vi "Lab Panel V4.88.vi"() -> ()   [LabVIEW 2013] (continued)
                n1776 = property on="O/I  LAB03-2" class="Bool (strict)"("DisabledEnum"=w3326) -> ()  [unwired: 2 in, 2 out]
                n1777 = Not(x=w3331) -> (.not. x?=w3332:bool)
                n1778 = Not(x=w3330) -> (.not. x?=w3333:bool)
                n1779 = Not(x=w3329) -> (.not. x?=w3334:bool)
                n1780 = property on="RESULT LAB05-2" class="Bool (strict)"("Visible"=w3332) -> ()  [unwired: 2 in, 2 out]
                n1781 = property on="RESULT LAB05-1" class="Bool (strict)"("Visible"=w3333) -> ()  [unwired: 2 in, 2 out]
                n1782 = Not(x=w3328) -> (.not. x?=w3335:bool)
                n1783 = property on="RESULT LAB04-2" class="Bool (strict)"("Visible"=w3334) -> ()  [unwired: 2 in, 2 out]
                n1784 = Not(x=w3327) -> (.not. x?=w3336:bool)
                n1785 = property on="RESULT LAB04-1" class="Bool (strict)"("Visible"=w3335) -> ()  [unwired: 2 in, 2 out]
                n1786 = property on="RESULT LAB03-2" class="Bool (strict)"("Visible"=w3336) -> ()  [unwired: 2 in, 2 out]
              }
              frame #2 {
                # "disable calibrate if any test running"
                n1787 = Or(x=w3359, y=w3358) -> (x .or. y?=w3352:bool)
                n1788 = Or(x=w3361, y=w3360) -> (x .or. y?=w3354:bool)
                n1789 = Or(x=w3365, y=w3364) -> (x .or. y?=w3356:bool)
                n1790 = Or(x=w3363, y=w3362) -> (x .or. y?=w3355:bool)
                n1791 = Or(x=w3367, y=w3366) -> (x .or. y?=w3357:bool)
                n1792 = Or(x=w3355, y=w3354) -> (x .or. y?=w3353:bool)
                n1793 = Or(x=w3357, y=w3356) -> (x .or. y?=w3351:bool)
                n1794 = Or(x=w3353, y=w3352) -> (x .or. y?=w3350:bool)
                n1795 = Or(x=w3351, y=w3350) -> (x .or. y?=w3349:bool)
                n1796 = case shown="False" w3349 {
                  tunnel: [0 2] -> w3348
                  frame False {
                  }
                  frame True {
                  }
                }
                n1797 = property on="JIG TEST" class="Clust (strict)"("DisabledEnum"=w3348) -> ()  [unwired: 2 in, 2 out]
                n1798 = property on="Network Directory" class="Path"("DisabledEnum"=w3348) -> ()  [unwired: 2 in, 2 out]
                n1799 = property on="MAIL SETTINGS" class="Clust (strict)"("DisabledEnum"=w3348) -> ()  [unwired: 2 in, 2 out]
                n1800 = property on="SET (cal)" class="Bool (strict)"("DisabledEnum"=w3348) -> ()  [unwired: 2 in, 2 out]
                n1801 = property on="ADMIN" class="Bool (strict)"("DisabledEnum"=0) -> ()  [unwired: 2 in, 2 out]
              }
            }
          }
          frame #8 {
            # "drive jigs"
            n1802 = stacked-sequence {
              frame #0 {
                # "jig on"
                n1803 = local read "jig cycle"() -> (w3375:dbl)
                n1804 = property on="JIG TEST" class="Clust (strict)"() -> ("DisabledEnum"=w3372:T16)  [unwired: 2 in, 2 out]
                n1805 = Equal?(x=w3372, y=2) -> (x = y?=w3371:bool)
                n1806 = Equal?(x=w3375, y=0) -> (x = y?=w3373:bool)
                n1807 = And(x=w3373, y=w3371) -> (x .and. y?=w3370:bool)
                n1808 = case shown="True" w3370 {
                  frame False {
                  }
                  frame True {
                    n1809 = local read "run lab01-1"() -> (w3386:bool)
                    n1810 = local read "run lab01-2"() -> (w3385:bool)
                    n1811 = local read "run lab02-1"() -> (w3384:bool)
                    n1812 = local read "run lab02-2"() -> (w3383:bool)
                    n1813 = local read "run lab03-1"() -> (w3382:bool)
                    n1814 = local read "run lab03-2"() -> (w3381:bool)
                    n1815 = local read "run lab04-1"() -> (w3380:bool)
                    n1816 = local read "run lab04-2"() -> (w3379:bool)
                    n1817 = local read "run lab05-1"() -> (w3378:bool)
                    n1818 = local read "run lab05-2"() -> (w3377:bool)
                    n1819 = local write "JIG LAB03-2"(w3381) -> ()
                    n1820 = local write "JIG LAB01-1"(w3386) -> ()
                    n1821 = local write "JIG LAB01-2"(w3385) -> ()
                    n1822 = local write "JIG LAB02-1"(w3384) -> ()
                    n1823 = local write "JIG LAB02-2"(w3383) -> ()
                    n1824 = local write "JIG LAB03-1"(w3382) -> ()
                    n1825 = local write "JIG LAB04-1"(w3380) -> ()
                    n1826 = local write "JIG LAB04-2"(w3379) -> ()
                    n1827 = local write "JIG LAB05-1"(w3378) -> ()
                    n1828 = local write "JIG LAB05-2"(w3377) -> ()
                  }
                }
              }
              frame #1 {
                # "jig off"
                n1829 = local read "jig cycle"() -> (w3393:dbl)
                n1830 = local read "on loops"() -> (w3392:dbl)
                n1831 = property on="JIG TEST" class="Clust (strict)"() -> ("DisabledEnum"=w3391:T16)  [unwired: 2 in, 2 out]
                n1832 = Equal?(x=w3391, y=2) -> (x = y?=w3389:bool)
                n1833 = Equal?(x=w3393, y=w3392) -> (x = y?=w3388:bool)
                n1834 = And(x=w3388, y=w3389) -> (x .and. y?=w3387:bool)
                n1835 = case shown="True" w3387 {
                  frame False {
                  }
                  frame True {
                    w3444 = FALSE
                    w3445 = TRUE
                    w3443 = 2
                    n1836 = local read "SELECT LAB05-2"() -> (w3434:T3)
                    n1837 = local read "SELECT LAB04-2"() -> (w3436:T3)
                    n1838 = local read "SELECT LAB04-1"() -> (w3437:T3)
                    n1839 = local read "SELECT LAB05-1"() -> (w3435:T3)
                    n1840 = local read "SELECT LAB03-2"() -> (w3438:T3)
                    n1841 = local read "SELECT LAB02-1"() -> (w3441:T3)
                    n1842 = local read "SELECT LAB03-1"() -> (w3439:T3)
                    n1843 = local read "SELECT LAB02-2"() -> (w3440:T3)
                    n1844 = local read "SELECT LAB01-2"() -> (w3442:T3)
                    n1845 = local read "run lab05-1"() -> (w3404:bool)
                    n1846 = local read "run lab05-2"() -> (w3403:bool)
                    n1847 = local read "SELECT LAB01-1"() -> (w3446:T3)
                    n1848 = local read "run lab04-2"() -> (w3405:bool)
                    n1849 = local read "run lab04-1"() -> (w3406:bool)
                    n1850 = local read "run lab01-1"() -> (w3422:bool)
                    n1851 = local read "run lab01-2"() -> (w3411:bool)
                    n1852 = local read "run lab03-2"() -> (w3407:bool)
                    n1853 = local read "run lab03-1"() -> (w3408:bool)
                    n1854 = local read "run lab02-1"() -> (w3410:bool)
                    n1855 = local read "run lab02-2"() -> (w3409:bool)
                    n1856 = Equal?(x=w3443, y=w3439) -> (x = y?=w3417:bool)
                    n1857 = Equal?(x=w3443, y=w3438) -> (x = y?=w3416:bool)
                    n1858 = Equal?(x=w3443, y=w3437) -> (x = y?=w3415:bool)
                    n1859 = Equal?(x=w3443, y=w3436) -> (x = y?=w3414:bool)
                    n1860 = Equal?(x=w3443, y=w3435) -> (x = y?=w3413:bool)
                    n1861 = Equal?(x=w3443, y=w3434) -> (x = y?=w3412:bool)
                    n1862 = Equal?(x=w3443, y=w3446) -> (x = y?=w3423:bool)
                    n1863 = Equal?(x=w3443, y=w3441) -> (x = y?=w3419:bool)
                    n1864 = Equal?(x=w3443, y=w3440) -> (x = y?=w3418:bool)
                    n1865 = Equal?(x=w3443, y=w3442) -> (x = y?=w3420:bool)
                    n1866 = And(x=w3414, y=w3405) -> (x .and. y?=w3396:bool)
                    n1867 = And(x=w3417, y=w3408) -> (x .and. y?=w3399:bool)
                    n1868 = And(x=w3415, y=w3406) -> (x .and. y?=w3397:bool)
                    n1869 = And(x=w3412, y=w3403) -> (x .and. y?=w3394:bool)
                    n1870 = And(x=w3418, y=w3409) -> (x .and. y?=w3400:bool)
                    n1871 = And(x=w3416, y=w3407) -> (x .and. y?=w3398:bool)
                    n1872 = And(x=w3413, y=w3404) -> (x .and. y?=w3395:bool)
                    n1873 = And(x=w3420, y=w3411) -> (x .and. y?=w3402:bool)
                    n1874 = And(x=w3423, y=w3422) -> (x .and. y?=w3421:bool)
                    n1875 = And(x=w3419, y=w3410) -> (x .and. y?=w3401:bool)
                    n1876 = Select(t=w3445, s=w3421, f=w3444) -> (s? t:f=w3424:bool)
                    n1877 = Select(t=w3445, s=w3402, f=w3444) -> (s? t:f=w3425:bool)
                    n1878 = Select(t=w3445, s=w3401, f=w3444) -> (s? t:f=w3426:bool)
                    n1879 = Select(t=w3445, s=w3400, f=w3444) -> (s? t:f=w3427:bool)
                    n1880 = Select(t=w3445, s=w3399, f=w3444) -> (s? t:f=w3428:bool)
                    n1881 = Select(t=w3445, s=w3398, f=w3444) -> (s? t:f=w3429:bool)
                    n1882 = Select(t=w3445, s=w3397, f=w3444) -> (s? t:f=w3430:bool)
                    n1883 = Select(t=w3445, s=w3396, f=w3444) -> (s? t:f=w3431:bool)
                    n1884 = Select(t=w3445, s=w3395, f=w3444) -> (s? t:f=w3432:bool)
                    n1885 = Select(t=w3445, s=w3394, f=w3444) -> (s? t:f=w3433:bool)
                    n1886 = local write "JIG LAB03-2"(w3429) -> ()
                    n1887 = local write "JIG LAB02-1"(w3426) -> ()
                    n1888 = local write "JIG LAB02-2"(w3427) -> ()
                    n1889 = local write "JIG LAB01-2"(w3425) -> ()
                    n1890 = local write "JIG LAB03-1"(w3428) -> ()
                    n1891 = local write "JIG LAB01-1"(w3424) -> ()
                    n1892 = local write "JIG LAB05-2"(w3433) -> ()
                    n1893 = local write "JIG LAB04-1"(w3430) -> ()
                    n1894 = local write "JIG LAB05-1"(w3432) -> ()
                    n1895 = local write "JIG LAB04-2"(w3431) -> ()
                  }
                }
              }
            }
          }
          frame #9 {
            # "enable  jig test output if no test busy"
            n1896 = property on="JIG TEST" class="Clust (strict)"() -> ("DisabledEnum"=w3449:T16)  [unwired: 2 in, 2 out]
            n1897 = Equal?(x=w3449, y=0) -> (x = y?=w3447:bool)
            n1898 = case shown="True" w3447 {
              frame False {
              }
              frame True {
                n1899 = local read "JIG TEST"() -> (w3460:T10)
                n1900 = Unbundle(w3460) -> ("LAB01-1"=w3459:bool, "LAB01-2"=w3458:bool, "LAB02-1"=w3457:bool, "LAB02-2"=w3456:bool, "LAB03-1"=w3455:bool, "LAB03-2"=w3454:bool, "LAB04-1"=w3453:bool, "LAB04-2"=w3452:bool, "LAB05-1"=w3451:bool, "LAB05-2"=w3450:bool)
                n1901 = local write "JIG LAB05-1"(w3451) -> ()
                n1902 = local write "JIG LAB05-2"(w3450) -> ()
                n1903 = local write "JIG LAB04-1"(w3453) -> ()
                n1904 = local write "JIG LAB04-2"(w3452) -> ()
                n1905 = local write "JIG LAB03-2"(w3454) -> ()
                n1906 = local write "JIG LAB01-1"(w3459) -> ()
                n1907 = local write "JIG LAB02-1"(w3457) -> ()
                n1908 = local write "JIG LAB03-1"(w3455) -> ()
                n1909 = local write "JIG LAB01-2"(w3458) -> ()
                n1910 = local write "JIG LAB02-2"(w3456) -> ()
              }
            }
          }
          frame #10 {
            # "drive digital output"
            n1911 = local read "O/I  LAB05-2"() -> (w3467:bool)
            n1912 = local read "O/I  LAB05-1"() -> (w3469:bool)
            n1913 = local read "JIG LAB05-2"() -> (w3466:bool)
            n1914 = local read "O/I  LAB04-2"() -> (w3471:bool)
            n1915 = local read "JIG LAB05-1"() -> (w3468:bool)
            n1916 = local read "JIG LAB04-2"() -> (w3470:bool)
            n1917 = local read "O/I  LAB03-1"() -> (w3476:bool)
            n1918 = local read "O/I  LAB04-1"() -> (w3472:bool)
            n1919 = local read "O/I  LAB02-1"() -> (w3480:bool)
            n1920 = local read "O/I  LAB02-2"() -> (w3478:bool)
            n1921 = local read "O/I  LAB03-2"() -> (w3474:bool)
            n1922 = local read "JIG LAB04-1"() -> (w3465:bool)
            n1923 = local read "JIG LAB03-2"() -> (w3473:bool)
            n1924 = local read "O/I  LAB01-2"() -> (w3482:bool)
            n1925 = local read "JIG LAB02-1"() -> (w3479:bool)
            n1926 = local read "JIG LAB02-2"() -> (w3477:bool)
            n1927 = local read "JIG LAB03-1"() -> (w3475:bool)
            n1928 = local read "O/I  LAB01-1"() -> (w3484:bool)
            n1929 = local read "JIG LAB01-2"() -> (w3481:bool)
            n1930 = local read "JIG LAB01-1"() -> (w3483:bool)
            n1931 = Build Array(w3471, w3470, w3469, w3468, w3467, w3466) -> (w3462:bool[])
            n1932 = Build Array(w3477, w3476, w3475, w3474, w3473, w3472, w3465) -> (w3463:bool[])
            n1933 = Build Array(w3484, w3483, w3482, w3481, w3480, w3479, w3478) -> (w3464:bool[])
            n1934 = local read "simulate"() -> (w3461:bool)
            n1935 = case shown="False" w3461 {
              tunnel: w3464 -> [w3487 _]
              tunnel: w3463 -> [w3486 _]
              tunnel: w3462 -> [w3485 _]
              frame False {
                n1936 = call "sub vi - Drive Relays All v6.vi"("Array #2"=w3485, "Array #1"=w3486, "Array #0"=w3487) -> ()  [unwired: 8 in, 1 out]
              }
              frame True {
              }
            }
          }
          frame #11 {
            # "get analog values"
            n1937 = local read "on loops"() -> (w3494:dbl)
            n1938 = local read "jig cycle"() -> (w3491:dbl)
            n1939 = Add(x=w3494, y=1) -> (x+y=w3492:dbl)
            n1940 = Equal?(x=w3491, y=1) -> (x = y?=w3488:bool)
            n1941 = Equal?(x=w3491, y=w3492) -> (x = y?=w3490:bool)
            n1942 = Or(x=w3488, y=w3490) -> (x .or. y?=w3489:bool)
            n1943 = global write "Global display 3.vi" "cycle O/F"(w3488) -> ()
            n1944 = case shown="True" w3489 {
              tunnel: w3488 -> [_ w3497]
              frame False {
              }
              frame True {
                n1945 = local read "simulate"() -> (w3500:bool)
                n1946 = case shown="False" w3500 {
                  tunnel: [w3510 errorcluster[] [] ("array ERROR")] -> w3508
                  tunnel: [w3517 0.3 ("Analog loop time")] -> w3507
                  tunnel: [w3516 dynamicdata[] [] ("array GRAPH")] -> w3506
                  tunnel: [w3515 w3519] -> w3505
                  tunnel: [w3514 w3519] -> w3504
                  tunnel: [w3513 w3519] -> w3503
                  tunnel: [w3512 w3519] -> w3502
                  tunnel: [w3511 w3519] -> w3501
                  tunnel: w3497 -> [_ w3525]
                  tunnel: [w3509 2.92] -> w3496
                  frame False {
                    n1947 = call "sub vi - Read Analog All v9.11.vi"() -> ("Analog loop time"=w3517:dbl, "array GRAPH"=w3516:dynamicdata[], "LAB01"=w3515:T26, "LAB02"=w3514:T27, "LAB03"=w3513:T28, "LAB04"=w3512:T29, "deg C"=w3509:dbl, "array ERROR"=w3510:errorcluster[], "LAB05"=w3511:T30)  [unwired: 7 in]
                  }
                  frame True {
                    n1948 = local read "ON amps"() -> (w3524:dbl)
                    n1949 = local read "OFF amps"() -> (w3523:dbl)
                    n1950 = local read "VOLTS"() -> (w3521:dbl)
                    n1951 = local read "PF"() -> (w3520:dbl)
                    n1952 = Select(t=w3524, s=w3525, f=w3523) -> (s? t:f=w3522:dbl)
                    n1953 = Bundle("OFF amps"=w3522, "VOLTS"=w3521, "PF"=w3520, "OFF amps"=w3522, "VOLTS"=w3521, "PF"=w3520) -> (w3519:T31)  [unwired: 1 in]
                  }
                }
                n1954 = local read "simulate"() -> (w3499:bool)
                n1955 = stacked-sequence {
                  tunnel: w3508 -> [w3533 _ _ _ _ _ _]
                  tunnel: w3507 -> [w3532 _ _ _ _ _ _]
                  tunnel: w3506 -> [w3529 _ _ _ _ _ _]
                  tunnel: w3505 -> [_ w3580 _ _ _ _ _]
                  tunnel: w3504 -> [_ _ w3587 _ _ _ _]
                  tunnel: w3503 -> [_ _ _ w3616 _ _ _]
                  tunnel: w3502 -> [_ _ _ _ w3643 _ _]
                  tunnel: w3501 -> [_ _ _ _ _ w3672 _]
                  tunnel: w3499 -> [_ w3558 w3586 w3614 w3642 w3670 w3696]
                  tunnel: T14 {"1  (A) cal"=1.0, "1 (V) cal"=1.0, "1 (PF) cal"=1.0, "1 (TL) cal"=1.0, "1 (TN) cal"=1.0, "2 (A) cal"=1.0, "2 (V) cal"=1.0, "2 (PF) cal"=1.0, "2 (TL) cal"=1.0, "2 (TN) cal"=1.0} ("CAL LAB01") -> [_ w3557 w3585 w3613 w3641 w3669 _]
                  tunnel: w3496 -> [_ _ _ _ _ _ w3695]
                  frame #0 {
                    n1956 = local write "AI"(TRUE) -> ()
                    n1957 = global write "Global 1.vi" "RATE(Hz)"("RATE (Hz)") -> ()
                    n1958 = global write "Global 1.vi" "SAMPLES"("SAMPLES") -> ()
                    n1959 = Index Array(array=w3529, index=6) -> (element=→"LAB04-1 (GRAPH)":dynamicdata)
                    n1960 = Index Array(array=w3529, index=7) -> (element=→"LAB04-2 (GRAPH)":dynamicdata)
                    n1961 = Index Array(array=w3529, index=9) -> (element=→"LAB05-2 (GRAPH)":dynamicdata)
                    n1962 = Index Array(array=w3529, index=8) -> (element=→"LAB05-1 (GRAPH)":dynamicdata)
                    n1963 = Index Array(array=w3529, index=5) -> (element=→"LAB03-2 (GRAPH)":dynamicdata)
                    n1964 = Index Array(array=w3529, index=0) -> (element=→"LAB01-1 (GRAPH)":dynamicdata)
                    n1965 = Index Array(array=w3529, index=1) -> (element=→"LAB01-2 (GRAPH)":dynamicdata)
                    n1966 = Index Array(array=w3529, index=2) -> (element=→"LAB02-1 (GRAPH)":dynamicdata)
                    n1967 = Index Array(array=w3529, index=3) -> (element=→"LAB02-2 (GRAPH)":dynamicdata)
                    n1968 = Index Array(array=w3529, index=4) -> (element=→"LAB03-1 (GRAPH)":dynamicdata)
                    "AI loop time" <- w3532
                    "Analog Error Array" <- w3533
                  }
                  frame #1 {
                    n1969 = case shown="False" w3558 {
                      tunnel: [w3581 w3582] -> w3579
                      tunnel: w3557 -> [_ w3582]
                      frame False {
                        n1970 = local read "CAL LAB01"() -> (w3581:T14)
                      }
                      frame True {
                      }
                    }
                    n1971 = Unbundle By Name(w3580) -> ("OFF amps"=w3578:dbl, "VOLTS"=w3577:dbl, "PF"=w3576:dbl, "OFF amps"=w3575:dbl, "VOLTS"=w3574:dbl, "PF"=w3573:dbl)
                    n1972 = Unbundle By Name(w3579) -> ("1  (A) cal"=w3572:dbl, "1 (V) cal"=w3571:dbl, "1 (PF) cal"=w3570:dbl, "2 (A) cal"=w3569:dbl, "2 (V) cal"=w3568:dbl, "2 (PF) cal"=w3567:dbl)  [unwired: 4 out]
                    n1973 = Multiply(x=w3578, y=w3572) -> (x*y=w3565:dbl)
                    n1974 = Multiply(x=w3577, y=w3571) -> (x*y=w3564:dbl)
                    n1975 = Multiply(x=w3576, y=w3570) -> (x*y=w3563:dbl)
                    n1976 = Multiply(x=w3575, y=w3569) -> (x*y=w3561:dbl)
                    n1977 = Multiply(x=w3574, y=w3568) -> (x*y=w3560:dbl)
                    n1978 = Multiply(x=w3573, y=w3567) -> (x*y=w3559:dbl)
                    n1979 = local read "SIG LAB01-1"() -> (w3566:T2)
                    n1980 = local read "SIG LAB01-2"() -> (w3562:T2)
                    n1981 = Bundle By Name(cluster=w3566, "AMPS"=w3565, "VOLTS"=w3564, "PF"=w3563) -> (w3556:T2)
                    n1982 = Bundle By Name(cluster=w3562, "AMPS"=w3561, "VOLTS"=w3560, "PF"=w3559) -> (w3555:T2)
                    n1983 = global write "Global display 1.vi" "SIG LAB01-2"(w3555) -> ()
                    n1984 = global write "Global display 1.vi" "SIG LAB01-1"(w3556) -> ()
                    n1985 = local write "SIG LAB01-2"(w3555) -> ()
                    n1986 = local write "SIG LAB01-1"(w3556) -> ()
                  }
                  frame #2 {
                    n1987 = Unbundle By Name(w3587) -> ("OFF amps"=w3607:dbl, "VOLTS"=w3606:dbl, "PF"=w3605:dbl, "OFF amps"=w3604:dbl, "VOLTS"=w3603:dbl, "PF"=w3602:dbl)
                    n1988 = case shown="True" w3586 {
                      tunnel: [w3609 w3610] -> w3608
                      tunnel: w3585 -> [_ w3610]
                      frame False {
                        n1989 = local read "CAL LAB02"() -> (w3609:T15)
                      }
                      frame True {
                      }
                    }
                    n1990 = Unbundle By Name(w3608) -> ("1  (A) cal"=w3601:dbl, "1 (V) cal"=w3600:dbl, "1 (PF) cal"=w3599:dbl, "2 (A) cal"=w3598:dbl, "2 (V) cal"=w3597:dbl, "2 (PF) cal"=w3596:dbl)  [unwired: 4 out]
                    n1991 = Multiply(x=w3607, y=w3601) -> (x*y=w3594:dbl)
                    n1992 = Multiply(x=w3606, y=w3600) -> (x*y=w3593:dbl)
                    n1993 = Multiply(x=w3605, y=w3599) -> (x*y=w3592:dbl)
                    n1994 = Multiply(x=w3604, y=w3598) -> (x*y=w3590:dbl)
                    n1995 = Multiply(x=w3603, y=w3597) -> (x*y=w3589:dbl)
                    n1996 = Multiply(x=w3602, y=w3596) -> (x*y=w3588:dbl)
                    n1997 = local read "SIG LAB02-1"() -> (w3595:T2)
                    n1998 = local read "SIG LAB02-2"() -> (w3591:T2)
                    n1999 = Bundle By Name(cluster=w3595, "AMPS"=w3594, "VOLTS"=w3593, "PF"=w3592) -> (w3584:T2)
                    n2000 = Bundle By Name(cluster=w3591, "AMPS"=w3590, "VOLTS"=w3589, "PF"=w3588) -> (w3583:T2)
                    n2001 = global write "Global display 1.vi" "SIG LAB02-1"(w3584) -> ()
                    n2002 = local write "SIG LAB02-2"(w3583) -> ()
                    n2003 = global write "Global display 1.vi" "SIG LAB02-2"(w3583) -> ()
                    n2004 = local write "SIG LAB02-1"(w3584) -> ()
                  }
                  frame #3 {
                    n2005 = Unbundle By Name(w3616) -> ("OFF amps"=w3635:dbl, "VOLTS"=w3634:dbl, "PF"=w3633:dbl, "OFF amps"=w3632:dbl, "VOLTS"=w3631:dbl, "PF"=w3630:dbl)
                    n2006 = case shown="True" w3614 {
                      tunnel: [w3637 w3638] -> w3636
                      tunnel: w3613 -> [_ w3638]
                      frame False {
                        n2007 = local read "CAL LAB03"() -> (w3637:T14)
                      }
                      frame True {
                      }
                    }
                    n2008 = Unbundle By Name(w3636) -> ("1  (A) cal"=w3629:dbl, "1 (V) cal"=w3628:dbl, "1 (PF) cal"=w3627:dbl, "2 (A) cal"=w3626:dbl, "2 (V) cal"=w3625:dbl, "2 (PF) cal"=w3624:dbl)  [unwired: 4 out]
                    n2009 = Multiply(x=w3635, y=w3629) -> (x*y=w3622:dbl)
                    n2010 = Multiply(x=w3634, y=w3628) -> (x*y=w3615:dbl)
                    n2011 = Multiply(x=w3633, y=w3627) -> (x*y=w3621:dbl)
                    n2012 = Multiply(x=w3632, y=w3626) -> (x*y=w3619:dbl)
                    n2013 = Multiply(x=w3631, y=w3625) -> (x*y=w3618:dbl)
                    n2014 = Multiply(x=w3630, y=w3624) -> (x*y=w3617:dbl)
                    n2015 = local read "SIG LAB03-1"() -> (w3623:T2)
                    n2016 = local read "SIG LAB03-2"() -> (w3620:T2)
                    n2017 = Bundle By Name(cluster=w3623, "AMPS"=w3622, "VOLTS"=w3615, "PF"=w3621) -> (w3612:T2)
                    n2018 = Bundle By Name(cluster=w3620, "AMPS"=w3619, "VOLTS"=w3618, "PF"=w3617) -> (w3611:T2)
                    n2019 = global write "Global display 1.vi" "SIG LAB03-1"(w3612) -> ()
                    n2020 = global write "Global display 1.vi" "SIG LAB03-2"(w3611) -> ()
                    n2021 = local write "SIG LAB03-2"(w3611) -> ()
                    n2022 = local write "SIG LAB03-1"(w3612) -> ()
                  }
                  frame #4 {
                    n2023 = Unbundle By Name(w3643) -> ("OFF amps"=w3663:dbl, "VOLTS"=w3662:dbl, "PF"=w3661:dbl, "OFF amps"=w3660:dbl, "VOLTS"=w3659:dbl, "PF"=w3658:dbl)
                    n2024 = case shown="False" w3642 {
                      tunnel: [w3665 w3666] -> w3664
                      tunnel: w3641 -> [_ w3666]
                      frame False {
                        n2025 = local read "CAL LAB04"() -> (w3665:T14)
                      }
                      frame True {
                      }
                    }
                    n2026 = Unbundle By Name(w3664) -> ("1  (A) cal"=w3657:dbl, "1 (V) cal"=w3656:dbl, "1 (PF) cal"=w3655:dbl, "2 (A) cal"=w3654:dbl, "2 (V) cal"=w3653:dbl, "2 (PF) cal"=w3652:dbl)  [unwired: 4 out]
                    n2027 = Multiply(x=w3663, y=w3657) -> (x*y=w3650:dbl)
                    n2028 = Multiply(x=w3662, y=w3656) -> (x*y=w3649:dbl)
                    n2029 = Multiply(x=w3661, y=w3655) -> (x*y=w3648:dbl)
                    n2030 = Multiply(x=w3660, y=w3654) -> (x*y=w3646:dbl)
                    n2031 = Multiply(x=w3659, y=w3653) -> (x*y=w3645:dbl)
                    n2032 = Multiply(x=w3658, y=w3652) -> (x*y=w3644:dbl)
                    n2033 = local read "SIG LAB04-1"() -> (w3651:T2)
                    n2034 = local read "SIG LAB04-2"() -> (w3647:T2)
                    n2035 = Bundle By Name(cluster=w3651, "AMPS"=w3650, "VOLTS"=w3649, "PF"=w3648) -> (w3640:T2)
                    n2036 = Bundle By Name(cluster=w3647, "AMPS"=w3646, "VOLTS"=w3645, "PF"=w3644) -> (w3639:T2)
                    n2037 = global write "Global display 1.vi" "SIG LAB04-2"(w3639) -> ()
                    n2038 = global write "Global display 1.vi" "SIG LAB04-1"(w3640) -> ()
                    n2039 = local write "SIG LAB04-2"(w3639) -> ()
                    n2040 = local write "SIG LAB04-1"(w3640) -> ()
                  }
                  frame #5 {
                    n2041 = Unbundle By Name(w3672) -> ("OFF amps"=w3691:dbl, "VOLTS"=w3671:dbl, "PF"=w3690:dbl, "OFF amps"=w3689:dbl, "VOLTS"=w3688:dbl, "PF"=w3687:dbl)
                    n2042 = case shown="False" w3670 {
                      tunnel: [w3693 w3694] -> w3692
                      tunnel: w3669 -> [_ w3694]
                      frame False {
                        n2043 = local read "CAL LAB05"() -> (w3693:T14)
                      }
                      frame True {
                      }
                    }
                    n2044 = Unbundle By Name(w3692) -> ("1  (A) cal"=w3686:dbl, "1 (V) cal"=w3685:dbl, "1 (PF) cal"=w3684:dbl, "2 (A) cal"=w3683:dbl, "2 (V) cal"=w3682:dbl, "2 (PF) cal"=w3681:dbl)  [unwired: 4 out]
                    n2045 = Multiply(x=w3691, y=w3686) -> (x*y=w3679:dbl)
                    n2046 = Multiply(x=w3671, y=w3685) -> (x*y=w3678:dbl)
                    n2047 = Multiply(x=w3690, y=w3684) -> (x*y=w3677:dbl)
                    n2048 = Multiply(x=w3689, y=w3683) -> (x*y=w3675:dbl)
                    n2049 = Multiply(x=w3688, y=w3682) -> (x*y=w3674:dbl)
                    n2050 = Multiply(x=w3687, y=w3681) -> (x*y=w3673:dbl)
                    n2051 = local read "SIG LAB05-1"() -> (w3680:T2)
                    n2052 = local read "SIG LAB05-2"() -> (w3676:T2)
                    n2053 = Bundle By Name(cluster=w3680, "AMPS"=w3679, "VOLTS"=w3678, "PF"=w3677) -> (w3668:T2)
                    n2054 = Bundle By Name(cluster=w3676, "AMPS"=w3675, "VOLTS"=w3674, "PF"=w3673) -> (w3667:T2)
                    n2055 = global write "Global display 1.vi" "SIG LAB05-1"(w3668) -> ()
                    n2056 = global write "Global display 1.vi" "SIG LAB05-2"(w3667) -> ()
                    n2057 = local write "SIG LAB05-2"(w3667) -> ()
                    n2058 = local write "SIG LAB05-1"(w3668) -> ()
                  }
                  frame #6 {
                    # "update ambient referance temperature"
                    n2059 = case shown="False" w3696 {
                      tunnel: [w3699 100.0] -> w3698
                      frame False {
                        n2060 = local read "TEMP REF cal"() -> (w3699:dbl)
                      }
                      frame True {
                      }
                    }
                    n2061 = local read "PANEL #"() -> (w3697:dbl)
                    n2062 = case shown="1" w3697 {
                      tunnel: w3698 -> [_ w3705]
                      tunnel: w3695 -> [_ w3704]
                      frame 0, Default {
                      }
                      frame 1 {
                        n2063 = Multiply(x=w3705, y=w3704) -> (x*y=w3703:dbl)
                        n2064 = Subtract(x=w3703, y=272) -> (x-y=w3701:dbl)
                        n2065 = local write "Ref deg C"(w3701) -> ()
                      }
                    }
                    "deg C (volts)" <- w3695
                  }
                }
              }
            }
          }
          frame #12 {
            # "save test data to file"
            n2066 = Get Date/Time In Seconds() -> (seconds since 1Jan1904=w3706:timestamp)
            "File Time Stamp" <- w3706
            n2067 = local read "on loops"() -> (w3725:dbl)
            n2068 = local read "jig cycle"() -> (w3722:dbl)
            n2069 = Format Date/Time String(time format string (%c)="%H:%M%:%S", seconds (now)=w3706) -> (date/time string=w3710:string)  [unwired: 1 in]
            n2070 = Add(x=w3725, y=2) -> (x+y=w3723:dbl)
            n2071 = Build Array(w3710) -> (w3709:string[])
            n2072 = Equal?(x=w3722, y=1) -> (x = y?=w3708:bool)
            n2073 = Equal?(x=w3722, y=w3723) -> (x = y?=w3707:bool)
            n2074 = stacked-sequence {
              tunnel: w3721 -> [w3731 _ _ _ _ _ _ _ _ _]
              tunnel: w3720 -> [_ w3807 _ _ _ _ _ _ _ _]
              tunnel: w3719 -> [_ _ w3887 _ _ _ _ _ _ _]
              tunnel: w3718 -> [_ _ _ w3967 _ _ _ _ _ _]
              tunnel: w3717 -> [_ _ _ _ w4047 _ _ _ _ _]
              tunnel: w3716 -> [_ _ _ _ _ w4127 _ _ _ _]
              tunnel: w3715 -> [_ _ _ _ _ _ w4207 _ _ _]
              tunnel: w3714 -> [_ _ _ _ _ _ _ w4287 _ _]
              tunnel: w3713 -> [_ _ _ _ _ _ _ _ w4367 _]
              tunnel: w3712 -> [_ _ _ _ _ _ _ _ _ w4447]
              tunnel: w3709 -> [w3730 w3811 w3891 w3971 w4051 w4131 w4211 w4291 w4371 w4451]
              tunnel: w3708 -> [w3729 w3810 w3890 w3970 w4050 w4130 w4210 w4290 w4370 w4450]
              tunnel: w3707 -> [w3728 w3809 w3889 w3969 w4049 w4129 w4209 w4289 w4369 w4449]
              tunnel: w3706 -> [w3727 w3808 w3888 w3968 w4048 w4128 w4208 w4288 w4368 w4448]
              frame #0 {
                n2075 = case shown="True" w3731 {
                  tunnel: w3730 -> [_ w3736]
                  tunnel: w3729 -> [_ w3735]
                  tunnel: w3728 -> [_ w3733]
                  tunnel: w3727 -> [_ w3732]
                  frame False {
                  }
                  frame True {
                    n2076 = local read "DISP LAB01-1"() -> (w3737:T4)
                    n2077 = local read "SIG LAB01-1"() -> (w3738:T2)
                    n2078 = local read "ON L01-1"() -> (w3734:cluster{"amps":dbl, "volts":dbl, "pf":dbl})
                    n2079 = Unbundle(w3738) -> ("AMPS"=w3744:dbl, "VOLTS"=w3742:dbl, "PF"=w3741:dbl, "Tmp Live"=w3740:dbl, "Tmp Neut"=w3743:dbl)
                    n2080 = Unbundle(w3737) -> ("CYCLE"=w3739:dbl)  [unwired: 2 out]
                    n2081 = stacked-sequence {
                      tunnel: w3744 -> [w3748 w3767]
                      tunnel: w3743 -> [_ w3766]
                      tunnel: w3742 -> [w3747 w3765]
                      tunnel: w3741 -> [w3746 w3764]
                      tunnel: w3740 -> [_ w3763]
                      tunnel: w3739 -> [_ w3762]
                      tunnel: w3736 -> [_ w3761]
                      tunnel: w3735 -> [w3749 _]
                      tunnel: w3734 -> [w3745 w3759]
                      tunnel: w3733 -> [_ w3760]
                      tunnel: w3732 -> [_ w3755]
                      frame #0 {
                        n2082 = case shown="True" w3749 {
                          tunnel: w3748 -> [_ w3754]
                          tunnel: w3747 -> [_ w3753]
                          tunnel: w3746 -> [_ w3752]
                          tunnel: w3745 -> [_ w3750]
                          frame False {
                          }
                          frame True {
                            n2083 = Bundle(cluster=w3750, "amps"=w3754, "volts"=w3753, "pf"=w3752) -> (w3751:cluster{"amps":dbl, "volts":dbl, "pf":dbl})
                            n2084 = local write "ON L01-1"(w3751) -> ()
                          }
                        }
                      }
                      frame #1 {
                        n2085 = Unbundle(w3759) -> ("amps"=w3758:dbl, "volts"=w3757:dbl, "pf"=w3756:dbl)
                        n2086 = case shown="True" w3760 {
                          tunnel: w3767 -> [_ w3768]
                          tunnel: w3766 -> [_ w3806]
                          tunnel: w3765 -> [_ _]
                          tunnel: w3764 -> [_ _]
                          tunnel: w3763 -> [_ w3805]
                          tunnel: w3762 -> [_ w3804]
                          tunnel: w3761 -> [_ w3772]
                          tunnel: w3758 -> [_ w3769]
                          tunnel: w3757 -> [_ w3801]
                          tunnel: w3756 -> [_ w3800]
                          tunnel: w3755 -> [_ w3770]
                          frame False {
                          }
                          frame True {
                            n2087 = local read "TDMS LAB01-1"() -> (w3803:refnum<k34>)
                            n2088 = Build Array(w3801) -> (w3797:dbl[])
                            n2089 = Build Array(w3800) -> (w3796:dbl[])
                            n2090 = Build Array(w3805) -> (w3795:dbl[])
                            n2091 = Build Array(w3806) -> (w3794:dbl[])
                            n2092 = Build Array(w3769) -> (w3799:dbl[])
                            n2093 = Build Array(w3768) -> (w3798:dbl[])
                            n2094 = Build Array(w3804) -> (w3793:dbl[])
                            n2095 = Build Array("AMPS ON", "AMPS OFF", "VOLTS", "PF", "TEMP Live", "TEMP Neut", "CYCLE") -> (w3777:string[])
                            n2096 = Bundle By Name("Y"=w3799, "t0"=w3770) -> (w3792:waveform(dbl))  [unwired: 1 in]
                            n2097 = Bundle By Name("Y"=w3798, "t0"=w3770) -> (w3791:waveform(dbl))  [unwired: 1 in]
                            n2098 = Bundle By Name("Y"=w3797, "t0"=w3770) -> (w3790:waveform(dbl))  [unwired: 1 in]
                            n2099 = Bundle By Name("Y"=w3796, "t0"=w3770) -> (w3789:waveform(dbl))  [unwired: 1 in]
                            n2100 = Bundle By Name("Y"=w3795, "t0"=w3770) -> (w3788:waveform(dbl))  [unwired: 1 in]
                            n2101 = Bundle By Name("Y"=w3794, "t0"=w3770) -> (w3787:waveform(dbl))  [unwired: 1 in]
                            n2102 = Bundle By Name("Y"=w3793, "t0"=w3770) -> (w3786:waveform(dbl))  [unwired: 1 in]
                            n2103 = Build Array(w3792, w3791, w3790, w3789, w3788, w3787, w3786) -> (w3785:waveform(dbl)[])
                            n2104 = TDMS Write(0:w3803, 5:"TEST VALUES", 7:w3777, 9:w3785) -> (4:w3776:refnum<k34>, 6:w3775:string, 15:w3774:errorcluster)  [unwired: 2 in, 1 out]
                            n2105 = TDMS Write(0:w3776, 5:w3775, 7:"TIME", 9:w3772, 11:w3774) -> (15:w3771:errorcluster)  [unwired: 1 in, 3 out]
                            n2106 = local write "data file error"(w3771) -> ()
                          }
                        }
                      }
                    }
                  }
                }
              }
              frame #1 {
                n2107 = case shown="True" w3807 {
                  tunnel: w3811 -> [_ w3816]
                  tunnel: w3810 -> [_ w3815]
                  tunnel: w3809 -> [_ w3813]
                  tunnel: w3808 -> [_ w3812]
                  frame False {
                  }
                  frame True {
                    n2108 = local read "DISP LAB01-2"() -> (w3817:T4)
                    n2109 = local read "SIG LAB01-2"() -> (w3818:T2)
                    n2110 = local read "ON L01-2"() -> (w3814:cluster{"amps":dbl, "volts":dbl, "pf":dbl})
                    n2111 = Unbundle(w3818) -> ("AMPS"=w3824:dbl, "VOLTS"=w3822:dbl, "PF"=w3821:dbl, "Tmp Live"=w3820:dbl, "Tmp Neut"=w3823:dbl)
                    n2112 = Unbundle(w3817) -> ("CYCLE"=w3819:dbl)  [unwired: 2 out]
                    n2113 = stacked-sequence {
                      tunnel: w3824 -> [w3828 w3847]
                      tunnel: w3823 -> [_ w3846]
                      tunnel: w3822 -> [w3827 w3845]
                      tunnel: w3821 -> [w3826 w3844]
                      tunnel: w3820 -> [_ w3843]
                      tunnel: w3819 -> [_ w3842]
                      tunnel: w3816 -> [_ w3841]
                      tunnel: w3815 -> [w3829 _]
                      tunnel: w3814 -> [w3825 w3839]
                      tunnel: w3813 -> [_ w3840]
                      tunnel: w3812 -> [_ w3835]
                      frame #0 {
                        n2114 = case shown="True" w3829 {
                          tunnel: w3828 -> [_ w3834]
                          tunnel: w3827 -> [_ w3833]
                          tunnel: w3826 -> [_ w3832]
                          tunnel: w3825 -> [_ w3830]
                          frame False {
                          }
                          frame True {
                            n2115 = Bundle(cluster=w3830, "amps"=w3834, "volts"=w3833, "pf"=w3832) -> (w3831:cluster{"amps":dbl, "volts":dbl, "pf":dbl})
                            n2116 = local write "ON L01-2"(w3831) -> ()
                          }
                        }
                      }
                      frame #1 {
                        n2117 = Unbundle(w3839) -> ("amps"=w3838:dbl, "volts"=w3837:dbl, "pf"=w3836:dbl)
                        n2118 = case shown="True" w3840 {
                          tunnel: w3847 -> [_ w3879]
                          tunnel: w3846 -> [_ w3886]
                          tunnel: w3845 -> [_ _]
                          tunnel: w3844 -> [_ _]
                          tunnel: w3843 -> [_ w3885]
                          tunnel: w3842 -> [_ w3884]
                          tunnel: w3841 -> [_ w3849]
                          tunnel: w3838 -> [_ w3881]
                          tunnel: w3837 -> [_ w3880]
                          tunnel: w3836 -> [_ w3878]
                          tunnel: w3835 -> [_ w3870]
                          frame False {
                          }
                          frame True {
                            n2119 = local read "TDMS LAB01-2"() -> (w3883:refnum<k34>)
                            n2120 = Build Array(w3880) -> (w3875:dbl[])
                            n2121 = Build Array(w3878) -> (w3874:dbl[])
                            n2122 = Build Array(w3885) -> (w3873:dbl[])
                            n2123 = Build Array(w3886) -> (w3872:dbl[])
                            n2124 = Build Array(w3881) -> (w3877:dbl[])
                            n2125 = Build Array(w3879) -> (w3876:dbl[])
                            n2126 = Build Array(w3884) -> (w3871:dbl[])
                            n2127 = Build Array("AMPS ON", "AMPS OFF", "VOLTS", "PF", "TEMP Live", "TEMP Neut", "CYCLE") -> (w3854:string[])
                            n2128 = Bundle By Name("Y"=w3877, "t0"=w3870) -> (w3869:waveform(dbl))  [unwired: 1 in]
                            n2129 = Bundle By Name("Y"=w3876, "t0"=w3870) -> (w3868:waveform(dbl))  [unwired: 1 in]
                            n2130 = Bundle By Name("Y"=w3875, "t0"=w3870) -> (w3867:waveform(dbl))  [unwired: 1 in]
                            n2131 = Bundle By Name("Y"=w3874, "t0"=w3870) -> (w3866:waveform(dbl))  [unwired: 1 in]
                            n2132 = Bundle By Name("Y"=w3873, "t0"=w3870) -> (w3865:waveform(dbl))  [unwired: 1 in]
                            n2133 = Bundle By Name("Y"=w3872, "t0"=w3870) -> (w3864:waveform(dbl))  [unwired: 1 in]
                            n2134 = Bundle By Name("Y"=w3871, "t0"=w3870) -> (w3863:waveform(dbl))  [unwired: 1 in]
                            n2135 = Build Array(w3869, w3868, w3867, w3866, w3865, w3864, w3863) -> (w3862:waveform(dbl)[])
                            n2136 = TDMS Write(0:w3883, 5:"TEST VALUES", 7:w3854, 9:w3862) -> (4:w3853:refnum<k34>, 6:w3852:string, 15:w3851:errorcluster)  [unwired: 2 in, 1 out]
                            n2137 = TDMS Write(0:w3853, 5:w3852, 7:"TIME", 9:w3849, 11:w3851) -> (15:w3848:errorcluster)  [unwired: 1 in, 3 out]
                            n2138 = local write "data file error"(w3848) -> ()
                          }
                        }
                      }
                    }
                  }
                }
              }
              frame #2 {
                n2139 = case shown="True" w3887 {
                  tunnel: w3891 -> [_ w3896]
                  tunnel: w3890 -> [_ w3895]
                  tunnel: w3889 -> [_ w3893]
                  tunnel: w3888 -> [_ w3892]
                  frame False {
                  }
                  frame True {
                    n2140 = local read "DISP LAB02-1"() -> (w3897:T4)
                    n2141 = local read "SIG LAB02-1"() -> (w3898:T2)
                    n2142 = local read "ON L02-1"() -> (w3894:cluster{"amps":dbl, "volts":dbl, "pf":dbl})
                    n2143 = Unbundle(w3898) -> ("AMPS"=w3904:dbl, "VOLTS"=w3902:dbl, "PF"=w3901:dbl, "Tmp Live"=w3900:dbl, "Tmp Neut"=w3903:dbl)
                    n2144 = Unbundle(w3897) -> ("CYCLE"=w3899:dbl)  [unwired: 2 out]
                    n2145 = stacked-sequence {
                      tunnel: w3904 -> [w3908 w3927]
                      tunnel: w3903 -> [_ w3926]
                      tunnel: w3902 -> [w3907 w3925]
                      tunnel: w3901 -> [w3906 w3924]
                      tunnel: w3900 -> [_ w3923]
                      tunnel: w3899 -> [_ w3922]
                      tunnel: w3896 -> [_ w3921]
                      tunnel: w3895 -> [w3909 _]
                      tunnel: w3894 -> [w3905 w3919]
                      tunnel: w3893 -> [_ w3920]
                      tunnel: w3892 -> [_ w3915]
                      frame #0 {
                        n2146 = case shown="True" w3909 {
                          tunnel: w3908 -> [_ w3914]
                          tunnel: w3907 -> [_ w3913]
                          tunnel: w3906 -> [_ w3912]
                          tunnel: w3905 -> [_ w3910]
                          frame False {
                          }
                          frame True {
                            n2147 = Bundle(cluster=w3910, "amps"=w3914, "volts"=w3913, "pf"=w3912) -> (w3911:cluster{"amps":dbl, "volts":dbl, "pf":dbl})
                            n2148 = local write "ON L02-1"(w3911) -> ()
                          }
                        }
                      }
                      frame #1 {
                        n2149 = Unbundle(w3919) -> ("amps"=w3918:dbl, "volts"=w3917:dbl, "pf"=w3916:dbl)
                        n2150 = case shown="True" w3920 {
                          tunnel: w3927 -> [_ w3959]
                          tunnel: w3926 -> [_ w3966]
                          tunnel: w3925 -> [_ _]
                          tunnel: w3924 -> [_ _]
                          tunnel: w3923 -> [_ w3965]
                          tunnel: w3922 -> [_ w3964]
                          tunnel: w3921 -> [_ w3929]
                          tunnel: w3918 -> [_ w3961]
                          tunnel: w3917 -> [_ w3960]
                          tunnel: w3916 -> [_ w3958]
                          tunnel: w3915 -> [_ w3950]
                          frame False {
                          }
                          frame True {
                            n2151 = local read "TDMS LAB02-1"() -> (w3963:refnum<k34>)
                            n2152 = Build Array(w3960) -> (w3955:dbl[])
                            n2153 = Build Array(w3958) -> (w3954:dbl[])
                            n2154 = Build Array(w3965) -> (w3953:dbl[])
                            n2155 = Build Array(w3966) -> (w3952:dbl[])
                            n2156 = Build Array(w3961) -> (w3957:dbl[])
                            n2157 = Build Array(w3959) -> (w3956:dbl[])
                            n2158 = Build Array(w3964) -> (w3951:dbl[])
                            n2159 = Build Array("AMPS ON", "AMPS OFF", "VOLTS", "PF", "TEMP Live", "TEMP Neut", "CYCLE") -> (w3934:string[])
                            n2160 = Bundle By Name("Y"=w3957, "t0"=w3950) -> (w3949:waveform(dbl))  [unwired: 1 in]
                            n2161 = Bundle By Name("Y"=w3956, "t0"=w3950) -> (w3948:waveform(dbl))  [unwired: 1 in]
                            n2162 = Bundle By Name("Y"=w3955, "t0"=w3950) -> (w3947:waveform(dbl))  [unwired: 1 in]
                            n2163 = Bundle By Name("Y"=w3954, "t0"=w3950) -> (w3946:waveform(dbl))  [unwired: 1 in]
                            n2164 = Bundle By Name("Y"=w3953, "t0"=w3950) -> (w3945:waveform(dbl))  [unwired: 1 in]
                            n2165 = Bundle By Name("Y"=w3952, "t0"=w3950) -> (w3944:waveform(dbl))  [unwired: 1 in]
                            n2166 = Bundle By Name("Y"=w3951, "t0"=w3950) -> (w3943:waveform(dbl))  [unwired: 1 in]
                            n2167 = Build Array(w3949, w3948, w3947, w3946, w3945, w3944, w3943) -> (w3942:waveform(dbl)[])
                            n2168 = TDMS Write(0:w3963, 5:"TEST VALUES", 7:w3934, 9:w3942) -> (4:w3933:refnum<k34>, 6:w3932:string, 15:w3931:errorcluster)  [unwired: 2 in, 1 out]
                            n2169 = TDMS Write(0:w3933, 5:w3932, 7:"TIME", 9:w3929, 11:w3931) -> (15:w3928:errorcluster)  [unwired: 1 in, 3 out]
                            n2170 = local write "data file error"(w3928) -> ()
                          }
                        }
                      }
                    }
                  }
                }
              }
              frame #3 {
                n2171 = case shown="True" w3967 {
                  tunnel: w3971 -> [_ w3976]
                  tunnel: w3970 -> [_ w3975]
                  tunnel: w3969 -> [_ w3973]
                  tunnel: w3968 -> [_ w3972]
                  frame False {
                  }
                  frame True {
                    n2172 = local read "DISP LAB02-2"() -> (w3977:T4)
                    n2173 = local read "SIG LAB02-2"() -> (w3978:T2)
                    n2174 = local read "ON L02-2"() -> (w3974:cluster{"amps":dbl, "volts":dbl, "pf":dbl})
                    n2175 = Unbundle(w3978) -> ("AMPS"=w3984:dbl, "VOLTS"=w3982:dbl, "PF"=w3981:dbl, "Tmp Live"=w3980:dbl, "Tmp Neut"=w3983:dbl)
                    n2176 = Unbundle(w3977) -> ("CYCLE"=w3979:dbl)  [unwired: 2 out]
                    n2177 = stacked-sequence {
                      tunnel: w3984 -> [w3988 w4007]
                      tunnel: w3983 -> [_ w4006]
                      tunnel: w3982 -> [w3987 w4005]
                      tunnel: w3981 -> [w3986 w4004]
                      tunnel: w3980 -> [_ w4003]
                      tunnel: w3979 -> [_ w4002]
                      tunnel: w3976 -> [_ w4001]
                      tunnel: w3975 -> [w3989 _]
                      tunnel: w3974 -> [w3985 w3999]
                      tunnel: w3973 -> [_ w4000]
                      tunnel: w3972 -> [_ w3995]
                      frame #0 {
                        n2178 = case shown="True" w3989 {
                          tunnel: w3988 -> [_ w3994]
                          tunnel: w3987 -> [_ w3993]
                          tunnel: w3986 -> [_ w3992]
                          tunnel: w3985 -> [_ w3990]
                          frame False {
                          }
                          frame True {
                            n2179 = Bundle(cluster=w3990, "amps"=w3994, "volts"=w3993, "pf"=w3992) -> (w3991:cluster{"amps":dbl, "volts":dbl, "pf":dbl})
                            n2180 = local write "ON L02-2"(w3991) -> ()
                          }
                        }
                      }
                      frame #1 {
                        n2181 = Unbundle(w3999) -> ("amps"=w3998:dbl, "volts"=w3997:dbl, "pf"=w3996:dbl)
                        n2182 = case shown="True" w4000 {
                          tunnel: w4007 -> [_ w4039]
                          tunnel: w4006 -> [_ w4046]
                          tunnel: w4005 -> [_ _]
                          tunnel: w4004 -> [_ _]
                          tunnel: w4003 -> [_ w4045]
                          tunnel: w4002 -> [_ w4044]
                          tunnel: w4001 -> [_ w4009]
                          tunnel: w3998 -> [_ w4041]
                          tunnel: w3997 -> [_ w4040]
                          tunnel: w3996 -> [_ w4038]
                          tunnel: w3995 -> [_ w4030]
                          frame False {
                          }
                          frame True {
                            n2183 = local read "TDMS LAB02-2"() -> (w4043:refnum<k34>)
                            n2184 = Build Array(w4040) -> (w4035:dbl[])
                            n2185 = Build Array(w4038) -> (w4034:dbl[])
                            n2186 = Build Array(w4045) -> (w4033:dbl[])
                            n2187 = Build Array(w4046) -> (w4032:dbl[])
